vi "set_query.vi"() -> ()   [LabVIEW 2020]
panel:
  out "read buffer":string
  out "return count 6":u32
  out "return count 5":u32
  out "error out 3":errorcluster
  out "return count 4":u32
  # "Change the range by double\n clicking the max value on the scale"
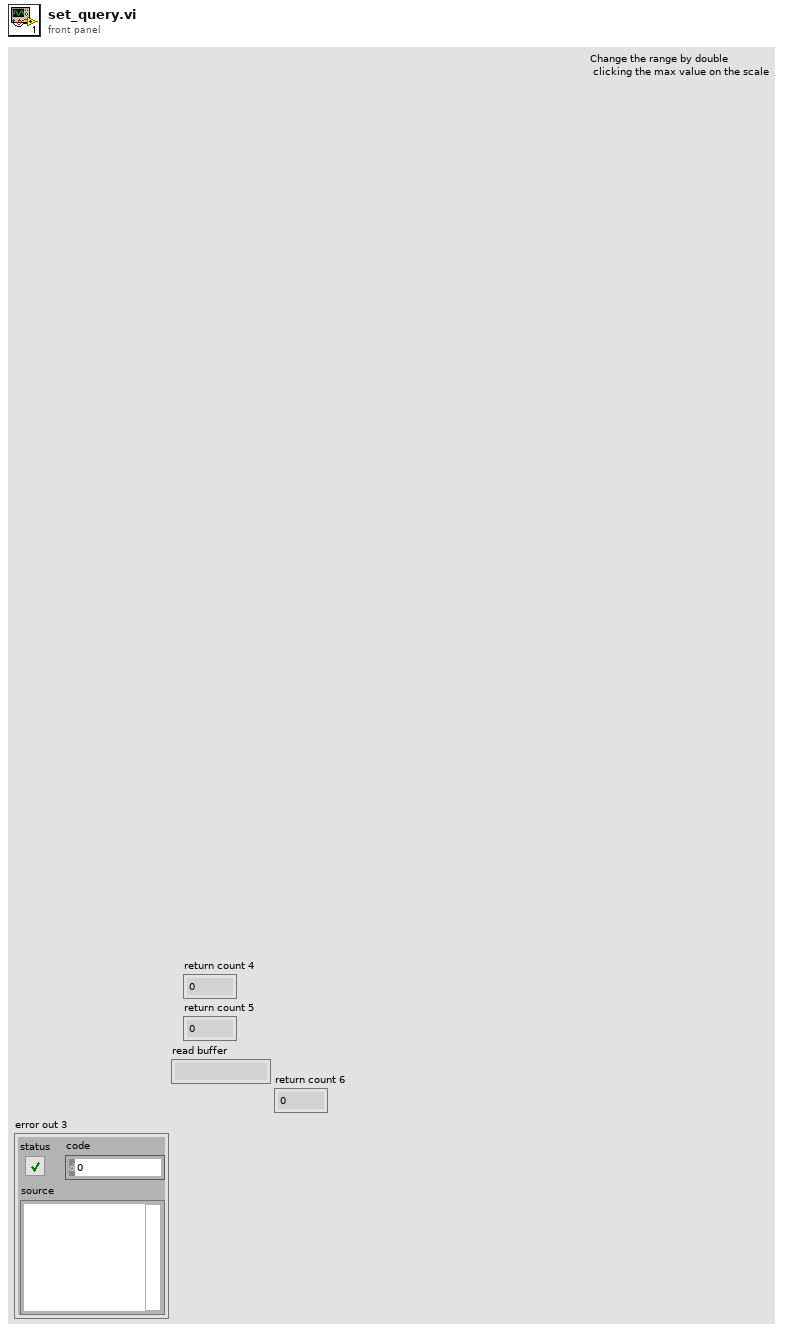
[diagram p1: front panel]
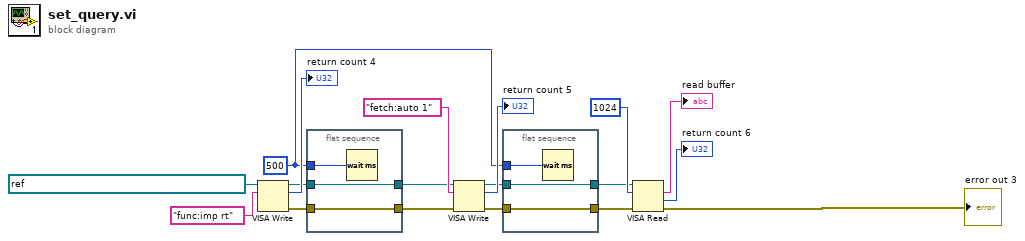
[diagram p0: block diagram]
diagram:
  w3 = u32 500 ("delay before read (ms)")
  n1 = VISA Write(VISA resource name=refnum<visa-resource-name> "USB0::0x0471::0x2515::482A16001::INSTR", write buffer="func:imp rt") -> (VISA resource name out=w11:refnum<visa-resource-name>, return count=→"return count 4":u32, error out=w10:errorcluster)  [unwired: 1 in]
  n2 = flat-sequence {
    tunnel: w10 -> [w20]
    tunnel: [w20] -> w8
    tunnel: w11 -> [w19]
    tunnel: [w19] -> w9
    tunnel: w3 -> [w21]
    frame #0 {
      n3 = Wait (ms)(milliseconds to wait=w21) -> ()  [unwired: 1 out]
    }
  }
  n4 = VISA Write(VISA resource name=w9, write buffer="fetch:auto 1", error in (no error)=w8) -> (VISA resource name out=w6:refnum<visa-resource-name>, return count=→"return count 5":u32, error out=w7:errorcluster)
  n5 = flat-sequence {
    tunnel: w7 -> [w24]
    tunnel: [w24] -> w4
    tunnel: w6 -> [w23]
    tunnel: [w23] -> w5
    tunnel: w3 -> [w22]
    frame #0 {
      n6 = Wait (ms)(milliseconds to wait=w22) -> ()  [unwired: 1 out]
    }
  }
  n7 = VISA Read(VISA resource name=w5, byte count=u32 1024, error in (no error)=w4) -> (read buffer=→"read buffer":string, return count=→"return count 6":u32, error out=→"error out 3":errorcluster)  [unwired: 1 out]
